vi "Filter.vi"(10 "SensorData":T1) -> (2 "Low Freq. A":T2)   [LabVIEW 2019]
doc: "This VI uses low-pass filter to get gravity acceleration."
uses:
  <vilib>/ptbypt/NI_PtbyPt.lvlib
  ROVsensorData.ctl
panel:
  # "This VI uses low-pass filter to get gravity acceleration."
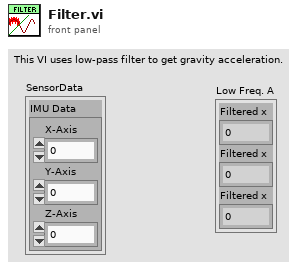
[diagram p1: front panel]
types:
  T1 = typedef "ROVsensorData.ctl" = cluster{"IMU Data":cluster{"X-Axis":dbl, "Y-Axis":dbl, "Z-Axis":dbl}}
  T2 = cluster{"Filtered x":dbl, "Filtered x":dbl, "Filtered x":dbl}
  T3 = cluster{"X-Axis":dbl, "Y-Axis":dbl, "Z-Axis":dbl}
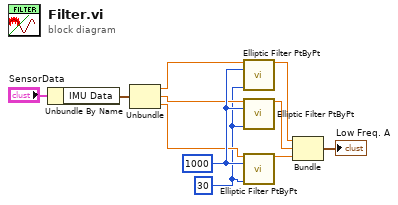
[diagram p0: block diagram]
diagram:
  w3 = 30
  w11 = 1000
  n1 = Unbundle By Name("SensorData") -> ("IMU Data"=w1:T3)
  n2 = Unbundle(w1) -> ("X-Axis"=w7:dbl, "Y-Axis"=w6:dbl, "Z-Axis"=w5:dbl)
  n3 = call <vilib>:"Elliptic Filter PtByPt.vi"("x"=w7, "sampling freq: fs"=w11, "low cutoff freq: fl"=w3) -> ("Filtered x"=w8:dbl)  [unwired: 11 in, 1 out]
  n4 = call <vilib>:"Elliptic Filter PtByPt.vi"("x"=w6, "sampling freq: fs"=w11, "low cutoff freq: fl"=w3) -> ("Filtered x"=w10:dbl)  [unwired: 11 in, 1 out]
  n5 = call <vilib>:"Elliptic Filter PtByPt.vi"("x"=w5, "sampling freq: fs"=w11, "low cutoff freq: fl"=w3) -> ("Filtered x"=w9:dbl)  [unwired: 11 in, 1 out]
  n6 = Bundle("Filtered x"=w8, "Filtered x"=w10, "Filtered x"=w9) -> (→"Low Freq. A":T2)  [unwired: 1 in]
